vi "Compute Nanotime Bin Size.vi"(8 "Error In":errorcluster, 9 "# Gates":i32, 11 "PicoQuant Data File Information":T1) -> (0 "Error Out":errorcluster, 2 "p (# native bins per user bin)":dbl, 3 "user bin size (Gate Step & Width) (s)":dbl format="%^#_6e")   [LabVIEW 2021, in "PTU Files.lvlib"]
uses:
  PTU Files.lvlib
  PicoQuant Data File Information.ctl
  PicoQuant File Information.ctl
  PicoQuant Software Information.ctl
  PicoQuant Remote Request Information.ctl
  PicoQuant Hardware Information.ctl
  PicoQuant Input Channels.ctl
  PicoQuant Markers.ctl
  PicoQuant Modules.ctl
  PicoQuant Router Channels.ctl
  PicoQuant Measurement Information.ctl
  PicoQuant Image Information.ctl
  PicoQuant Results Format.ctl
  PicoQuant Measurement Results.ctl
panel:
  out "T (from SYNC rate)":dbl format="%^#_6e"
  out "T/d (# native bins per laser period)":dbl
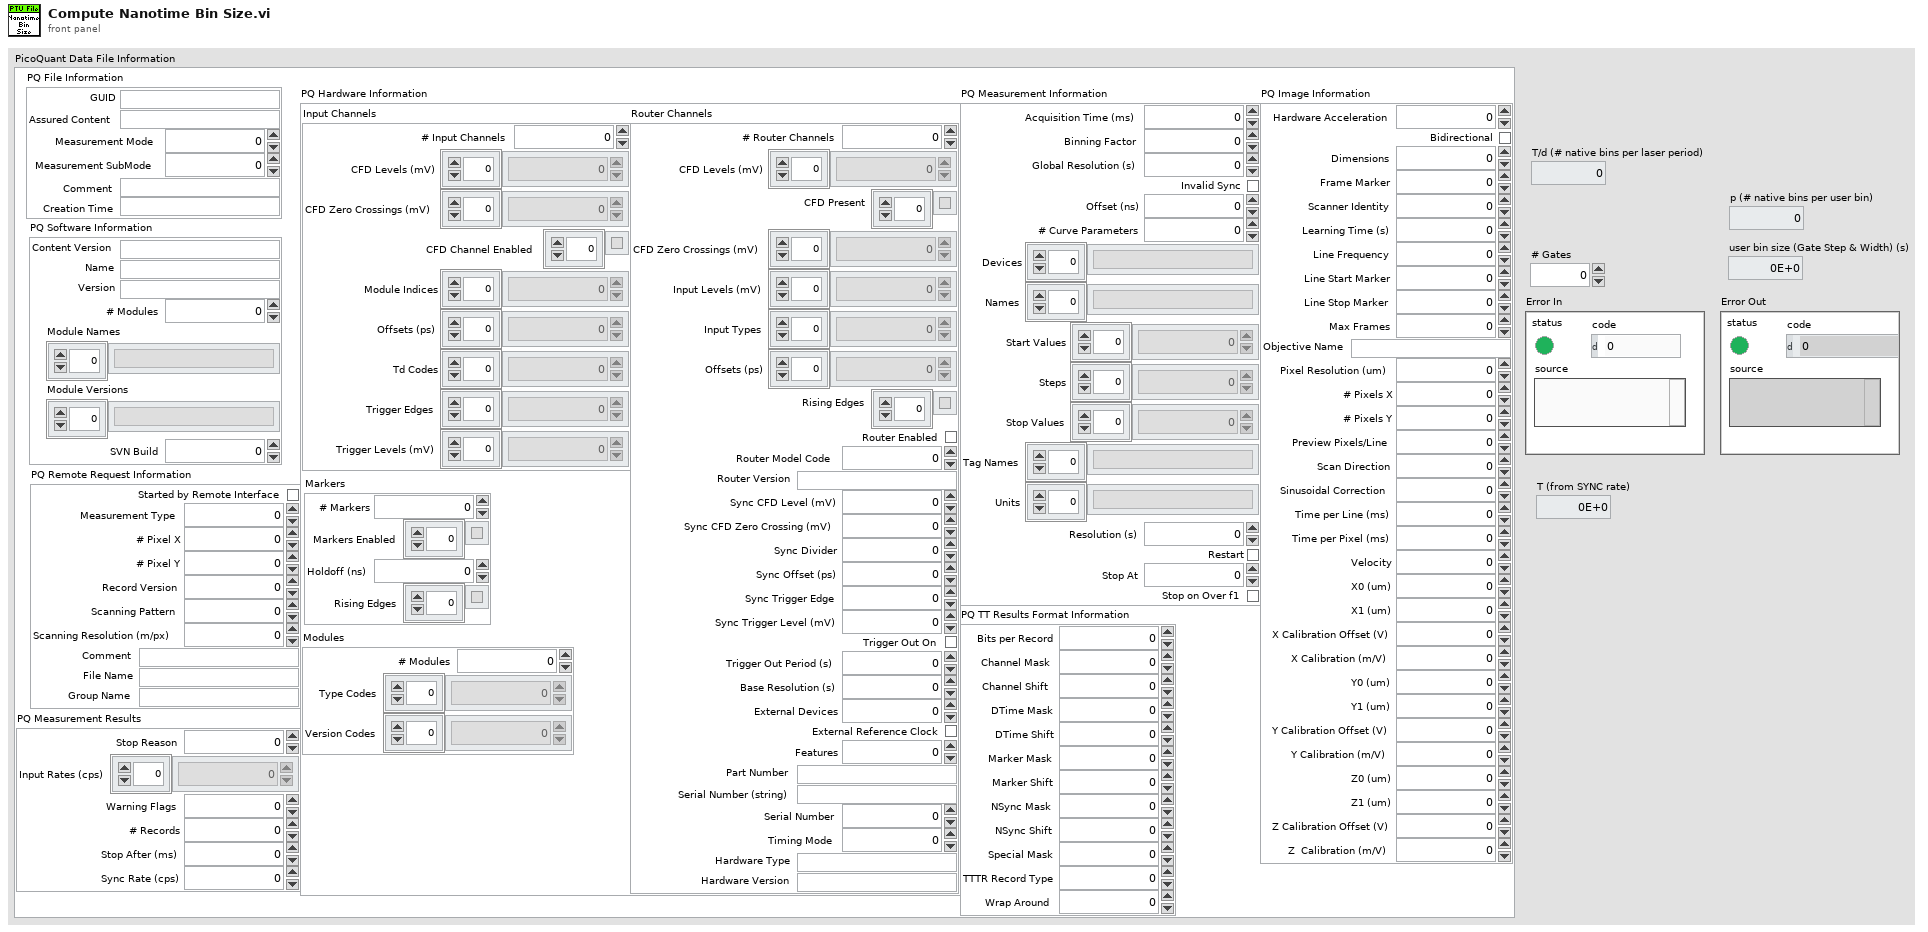
[diagram p1: front panel]
types:
  T1 = typedef "PTU Files.lvlib/PicoQuant Data File Information.ctl" = cluster{"PQ File Information":T2, "PQ Software Information":T3, "PQ Remote Request Information":T4, "PQ Hardware Information":T5, "PQ Measurement Information":T10, "PQ Image Information":T11, "PQ TT Results Format Information":T12, "PQ Measurement Results":T13}
  T2 = typedef "PTU Files.lvlib/PicoQuant File Information.ctl" = cluster{"GUID":string, "Assured Content":string, "Measurement Mode":i64, "Measurement SubMode":i64, "Comment":string, "Creation Time":string}
  T3 = typedef "PTU Files.lvlib/PicoQuant Software Information.ctl" = cluster{"Content Version":string, "Name":string, "Version":string, "# Modules":i64, "Module Names":string[], "Module Versions":string[], "SVN Build":i64}
  T4 = typedef "PTU Files.lvlib/PicoQuant Remote Request Information.ctl" = cluster{"Started by Remote Interface":bool, "Measurement Type":i64, "# Pixel X":i64, "# Pixel Y":i64, "Record Version":i64, "Scanning Pattern":i64, "Scanning Resolution (m/px)":dbl, "Comment":string, "File Name":string, "Group Name":string}
  T5 = typedef "PTU Files.lvlib/PicoQuant Hardware Information.ctl" = cluster{"Input Channels":T6, "Markers":T7, "Modules":T8, "Router Channels":T9}
  T6 = typedef "PTU Files.lvlib/PicoQuant Input Channels.ctl" = cluster{"# Input Channels":i64, "CFD Levels (mV)":i64[], "CFD Zero Crossings (mV)":i64[], "CFD Channel Enabled":bool[], "Module Indices":i64[], "Offsets (ps)":i64[], "Td Codes":i64[], "Trigger Edges":i64[], "Trigger Levels (mV)":i64[]}
  T7 = typedef "PTU Files.lvlib/PicoQuant Markers.ctl" = cluster{"# Markers":i64, "Markers Enabled":bool[], "Holdoff (ns)":i64, "Rising Edges":bool[]}
  T8 = typedef "PTU Files.lvlib/PicoQuant Modules.ctl" = cluster{"# Modules":i64, "Type Codes":i64[], "Version Codes":i64[]}
  T9 = typedef "PTU Files.lvlib/PicoQuant Router Channels.ctl" = cluster{"# Router Channels":i64, "CFD Levels (mV)":i64[], "CFD Present":bool[], "CFD Zero Crossings (mV)":i64[], "Input Levels (mV)":i64[], "Input Types":i64[], "Offsets (ps)":i64[], "Rising Edges":bool[], "Router Enabled":bool, "Router Model Code":i64, "Router Version":string, "Sync CFD Level (mV)":i64, "Sync CFD Zero Crossing (mV)":i64, "Sync Divider":i64, "Sync Offset (ps)":i64, "Sync Trigger Edge":i64, "Sync Trigger Level (mV)":i64, "Trigger Out On":bool, "Trigger Out Period (s)":dbl, "Base Resolution (s)":dbl, "External Devices":i64, "External Reference Clock":bool, "Features":u64, "Part Number":string, "Serial Number (string)":string, "Serial Number":i64, "Timing Mode":i64, "Hardware Type":string, "Hardware Version":string}
  T10 = typedef "PTU Files.lvlib/PicoQuant Measurement Information.ctl" = cluster{"Acquisition Time (ms)":i64, "Binning Factor":i64, "Global Resolution (s)":dbl, "Invalid Sync":bool, "Offset (ns)":u64, "# Curve Parameters":u64, "Devices":string[], "Names":string[], "Start Values":dbl[], "Steps":dbl[], "Stop Values":dbl[], "Tag Names":string[], "Units":string[], "Resolution (s)":dbl, "Restart":bool, "Stop At":u64, "Stop on Over f1":bool}
  T11 = typedef "PTU Files.lvlib/PicoQuant Image Information.ctl" = cluster{"Hardware Acceleration":i64, "Bidirectional":bool, "Dimensions":i64, "Frame Marker":i64, "Scanner Identity":i64, "Learning Time (s)":i64, "Line Frequency":dbl, "Line Start Marker":i64, "Line Stop Marker":i64, "Max Frames":i64, "Objective Name":string, "Pixel Resolution (um)":dbl, "# Pixels X":i64, "# Pixels Y":i64, "Preview Pixels/Line":i64, "Scan Direction":i64, "Sinusoidal Correction":i64, "Time per Line (ms)":dbl, "Time per Pixel (ms)":i64, "Velocity":i64, "X0 (um)":dbl, "X1 (um)":dbl, "X Calibration Offset (V)":dbl, "X Calibration (m/V)":dbl, "Y0 (um)":dbl, "Y1 (um)":dbl, "Y Calibration Offset (V)":dbl, "Y Calibration (m/V)":dbl, "Z0 (um)":dbl, "Z1 (um)":dbl, "Z Calibration Offset (V)":dbl, "Z  Calibration (m/V)":dbl}
  T12 = typedef "PTU Files.lvlib/PicoQuant Results Format.ctl" = cluster{"Bits per Record":i64, "Channel Mask":i64, "Channel Shift ":i64, "DTime Mask":i64, "DTime Shift":i64, "Marker Mask":i64, "Marker Shift":i64, "NSync Mask":i64, "NSync Shift":i64, "Special Mask":i64, "TTTR Record Type":i64, "Wrap Around":i64}
  T13 = typedef "PTU Files.lvlib/PicoQuant Measurement Results.ctl" = cluster{"Stop Reason":i64, "Input Rates (cps)":i64[], "Warning Flags":u64, "# Records":i64, "Stop After (ms)":i64, "Sync Rate (cps)":i64}
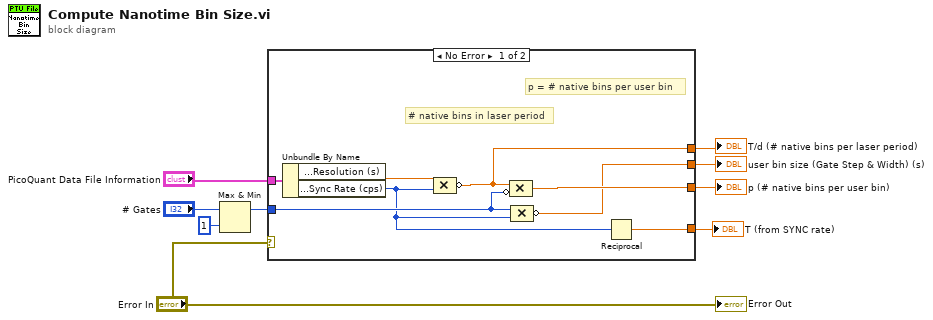
[diagram p0: block diagram]
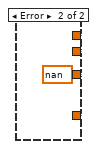
[diagram p2: hidden frame]
diagram:
  n1 = Max & Min(x="# Gates", y=1) -> (max(x,y)=w2:i32)  [unwired: 1 out]
  n2 = case shown="No Error" "Error In" {
    tunnel: "PicoQuant Data File Information" -> [w17 _]
    tunnel: [w10 w18] -> w8
    tunnel: [w15 w18] -> w5
    tunnel: w2 -> [w12 _]
    tunnel: [w14 w18] -> w6
    tunnel: [w13 w18] -> w3
    frame No Error {
      # "p = # native bins per user bin"
      # "# native bins in laser period"
      n3 = Unbundle By Name(w17) -> ("PQ Measurement Information.Resolution (s)"=w16:dbl, "PQ Measurement Results.Sync Rate (cps)"=w11:i64)
      n4 = Compound Arithmetic op=MULTIPLY(w16, w11) -> (invert w14:dbl)
      n5 = Compound Arithmetic op=MULTIPLY(w14, invert w12) -> (w15:dbl)
      n6 = Compound Arithmetic op=MULTIPLY(w12, w11) -> (invert w10:dbl)
      n7 = Reciprocal(x=w11) -> (1/x=w13:dbl)
    }
    frame Error {
      w18 = nan
    }
  }
  "user bin size (Gate Step & Width) (s)" <- w8
  "p (# native bins per user bin)" <- w5
  "T/d (# native bins per laser period)" <- w6
  "T (from SYNC rate)" <- w3
  "Error Out" <- "Error In"
